vi "Exemple - SyncSum.vi"() -> ()   [LabVIEW 2016]
uses:
  Library/DemoSkeleton/DemoSkeleton.lvlib
panel:
  out "Sum":i32
  in  "B":i32=2
  in  "A":i32=1
  # "+"
  # "="
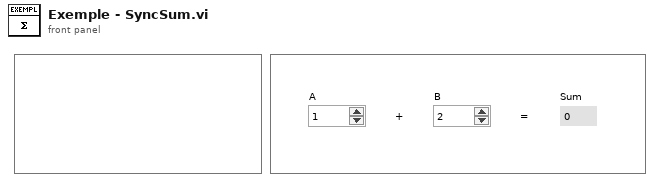
[diagram p1: front panel]
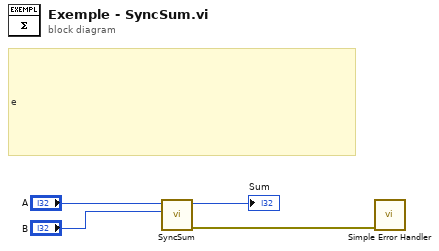
[diagram p0: block diagram]
diagram:
  # "e"
  n1 = call "SyncSum.vi"("B"="B", "A"="A") -> ("error out"=w2:errorcluster, "Sum"=→"Sum":i32)  [unwired: 8 in]
  n2 = call <vilib>:"Simple Error Handler.vi"("error in (no error)"=w2) -> ()  [unwired: 4 in, 5 out]
